vi "PPMS Monitor and Control.vi"() -> ()   [LabVIEW 2016, in "instrument.PPMS2.lvclass"]
doc: "This VI will launch the PPMS 2 Instrument backend that will contunously monitor the state of the instrument and log to the DSC. The user has the option of launching a user interface (default) or allowing the backend to run headless. Run \"Launch PPMS2 UI.vi\" here or on a different computer to have a remote user interface. You can also use the APIs like \"Get Temperturature\" interact programmatically with the PPMS 2 Instrument backend."
uses:
  instrument.PPMS2.lvclass
  <vilib>/JKI/JKI SMO/SMO/Typedefs/SMOState --Enum.ctl
  C:/Program Files (x86)/National Instruments/LabVIEW 2016/vi.lib/JKI/JKI SMO/SMO/SMO.lvclass
  instrument.PPMS2 UI/Instrument.PPMS2 UI.lvclass
  C:/Program Files (x86)/National Instruments/LabVIEW 2016/vi.lib/JKI/JKI SMO/SMO.UI/SMO.UI.lvclass
  <vilib>/JKI/JKI SMO/SMO/SMO.lvclass
  <vilib>/JKI/JKI SMO/SMO.UI/SMO.UI.lvclass
panel:
  in  "Start UI?":bool=TRUE
  in  "Stop":bool=TRUE
  in  "Start":bool=TRUE
  in  "Splash Status":string="Push Start to Start..." caption="String"
  out "UI SMO State":T1=enum."Stopped"
  out "SMO State":T1
  out "error out":errorcluster
  # "PPMS Monitor and Control.vi"
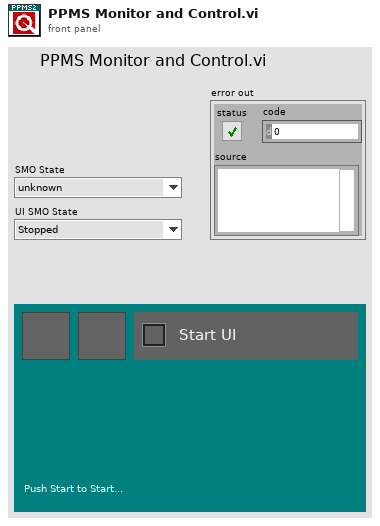
[diagram p1: front panel]
types:
  T1 = typedef "SMO.lvclass/SMOState --Enum.ctl" = enum16{"unknown", "Created", "Started", "Stopped"}
  T2 = enum32{"Invalid", "Standard", "Closed", "Hidden", "Minimized", "Maximized"}
  T3 = typedef "SMO.lvclass/Public Events.ctl" = cluster{"Error":refnum<user-event>, "State":refnum<user-event>, "Reserve State":refnum<user-event>}
  T4 = cluster{"Event Registration Refnum":refnum<event-registration>, "Event Registration Refnum":refnum<event-registration>}
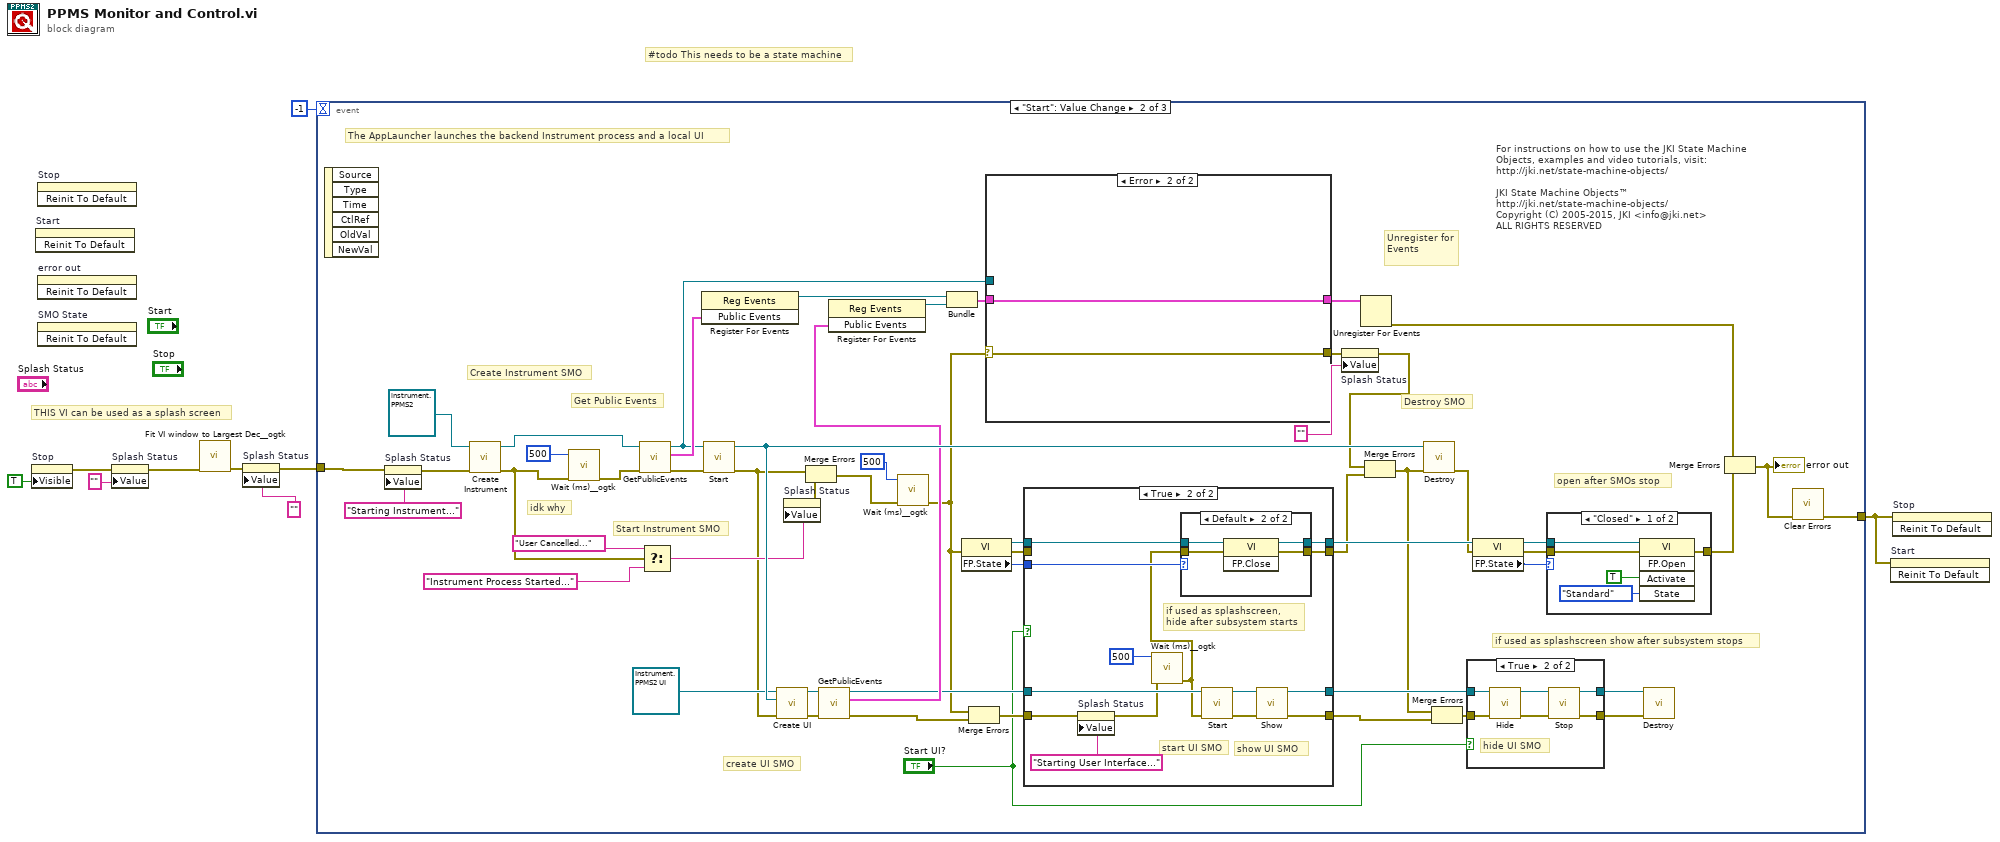
[diagram p0: block diagram]
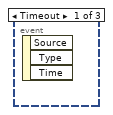
[diagram p2: hidden frame]
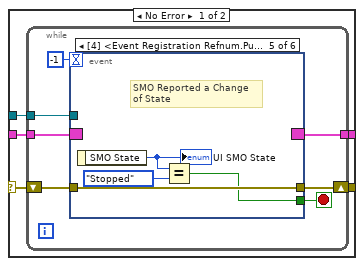
[diagram p3: hidden frame]
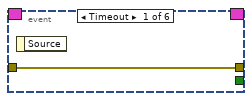
[diagram p4: hidden frame]
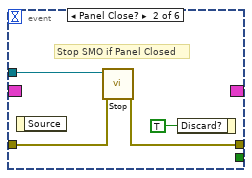
[diagram p5: hidden frame]
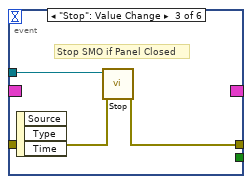
[diagram p6: hidden frame]
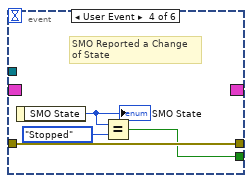
[diagram p7: hidden frame]
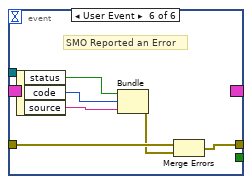
[diagram p8: hidden frame]
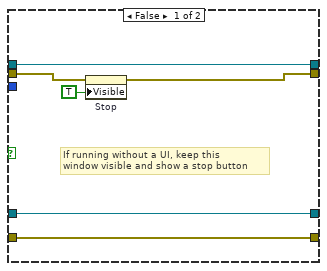
[diagram p10: hidden frame]
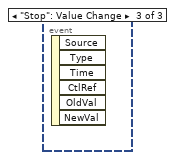
[diagram p13: hidden frame]
diagram:
  # "#todo This needs to be a state machine"
  # "THIS VI can be used as a splash screen"
  n1 = property on="Stop" class="Bool (strict)"("Visible"=TRUE) -> (error out=w7:errorcluster)  [unwired: 2 in, 1 out]
  n2 = invoke on="Start" class="Bool (strict)" method="Reinit To Default"() -> ()  [unwired: 3 in, 3 out]
  n3 = invoke on="Stop" class="Bool (strict)" method="Reinit To Default"() -> ()  [unwired: 3 in, 3 out]
  n4 = invoke on="error out" class="Clust (strict)" method="Reinit To Default"() -> ()  [unwired: 3 in, 3 out]
  n5 = invoke on="SMO State" class="Enum (strict)" method="Reinit To Default"() -> ()  [unwired: 3 in, 3 out]
  n6 = property on="Splash Status" class="Str"(error in=w7, "Value"="" ("Splash Status")) -> (error out=w9:errorcluster)  [unwired: 1 in, 1 out]
  n7 = call <userlib>:"Fit VI window to Largest Dec__ogtk.vi"("error in (no error)"=w9) -> ("error out"=w4:errorcluster)  [unwired: 5 in, 1 out]
  n8 = property on="Splash Status" class="Str"(error in=w4, "Value"="" ("Splash Status")) -> (error out=w3:errorcluster)  [unwired: 1 in, 1 out]
  n9 = event shown="[1] \"Start\": Value Change" {
    selector: _ -> [_ _ _]
    dyn-events: _ -> [_ _ _]
    timeout: -1 -> [_ _ _]
    tunnel: w3 -> [_ w21 _]
    tunnel: [_ w17 _] -> w1
    event Timeout {
      n10 = event-data() -> ()  [unwired: 1 in, 3 out]
    }
    event "Start": Value Change {
      # "idk why"
      # "open after SMOs stop"
      # "create UI SMO"
      # "if used as splashscreen show after subsystem stops"
      # "The AppLauncher launches the backend Instrument process and a local UI"
      # "Get Public Events"
      # "Start Instrument SMO"
      # "Destroy SMO"
      # "Create Instrument SMO"
      # "Unregister for Events"
      # "For instructions on how to use the JKI State Machine Objects, examples and video tutorials, visit:\nhttp://jki.net/state-machine-objects/\n\nJKI State Machine Objects™\nhttp://jki.net/state-machine-objects/\nCopyright (C) 2005-2015, JKI <info@jki.net>\nALL RIGHTS RESERVED"
      n11 = event-data() -> ()  [unwired: 1 in, 6 out]
      n12 = property on="Splash Status" class="Str"(error in=w21, "Value"="Starting Instrument..." ("Splash Status")) -> (error out=w30:errorcluster)  [unwired: 1 in, 1 out]
      n13 = call-dynamic "Create Instrument.vi"("error in (no error)"=w30, "Instrument in"=refnum<class "instrument.PPMS2.lvclass"> refnum ("SMO.Template.lvclass")) -> ("error out"=w16:errorcluster, "Instrument out"=w31:refnum<class "instrument.PPMS2.lvclass">)  [unwired: 8 in]
      n14 = call <userlib>:"Wait (ms)__ogtk.vi"("error in (no error)"=w16, "milliseconds to wait"=u32 500) -> ("error out"=w33:errorcluster)  [unwired: 8 in, 1 out]
      n15 = call <vilib>:"GetPublicEvents.vi"("error in (no error)"=w33, "SMO"=w31) -> ("error out"=w59:errorcluster, "Public Events"=w61:T3, "SMO out"=w60:refnum<class "instrument.PPMS2.lvclass">)  [unwired: 7 in]
      n16 = Select(t="User Cancelled...", s=w16, f="Instrument Process Started..." ("Splash Status")) -> (s? t:f=w15:string)
      n17 = register-events(w61) -> (reference out=w19:refnum<event-registration>)  [unwired: 2 in, 1 out]
      n18 = call <vilib>:"Start.vi"("error in (no error)"=w59, "SMO"=w60) -> ("error out"=w14:errorcluster, "SMO out"=w53:refnum<class "instrument.PPMS2.lvclass">)  [unwired: 8 in]
      n19 = call "Create UI.vi"("error in (no error)"=w14, "instrument.PPMS2"=w53, "Instrument.PPMS2 UI"=refnum<class "Instrument.PPMS2 UI.lvclass"> refnum ("SR7220 UI.lvclass")) -> ("error out"=w51:errorcluster, "Instrument.PPMS2 UI out"=w50:refnum<class "Instrument.PPMS2 UI.lvclass">)  [unwired: 7 in]
      n20 = property on="Splash Status" class="Str"("Value"=w15) -> (error out=w13:errorcluster)  [unwired: 2 in, 1 out]
      n21 = Merge Errors(w14, w13) -> (w12:errorcluster)
      n22 = call <vilib>:"GetPublicEvents.vi"("error in (no error)"=w51, "SMO"=w50) -> ("error out"=w44:errorcluster, "Public Events"=w49:T3, "SMO out"=w45:refnum<class "Instrument.PPMS2 UI.lvclass">)  [unwired: 7 in]
      n23 = register-events(w49) -> (reference out=w52:refnum<event-registration>)  [unwired: 2 in, 1 out]
      n24 = call <userlib>:"Wait (ms)__ogtk.vi"("error in (no error)"=w12, "milliseconds to wait"=u32 500) -> ("error out"=w18:errorcluster)  [unwired: 8 in, 1 out]
      n25 = Bundle("Event Registration Refnum"=w19, "Event Registration Refnum"=w52) -> (w54:T4)  [unwired: 1 in]
      n26 = property class="VI"(error in=w18) -> (reference out=w39:refnum<vi>, error out=w40:errorcluster, "FP.State"=w38:T2)  [unwired: 1 in]
      n27 = Merge Errors(w18, w44) -> (w48:errorcluster)
      n28 = case shown="Error" w18 {
        selector: w18 -> [w64 w99]
        tunnel: [w68 w98] -> w63
        tunnel: w60 -> [w67 _]
        tunnel: w54 -> [w66 w98]
        tunnel: [w65 w99] -> w27
        frame No Error {
          n29 = while {
            shift-right: [w74] -> w65
            shift-left: w64 -> [w73]
            tunnel: w66 -> [w72]
            tunnel: [w71] -> w68
            tunnel: w67 -> [w70]
            stop <- w75 stop-if-true
            n30 = event shown="[4] <Event Registration Refnum.Public Events.State>: User Event" {
              selector: w72 -> [_ _ _ _ _ _]
              dyn-events: [_ _ _ _ _ _] -> w71
              timeout: -1 -> [_ _ _ _ _ _]
              tunnel: [_ _ _ w84 w88 _] -> w75
              tunnel: w70 -> [_ w80 w83 _ _ _]
              tunnel: [w76 w79 w82 w87 w91 w92] -> w74
              tunnel: w73 -> [w76 w78 w81 w87 w91 w94]
              event Timeout {
                n31 = event-data() -> ()  [unwired: 1 in, 1 out]
              }
              event Panel Close? {
                # "Stop SMO if Panel Closed"
                n32 = event-data() -> ()  [unwired: 1 in, 1 out]
                n33 = call <vilib>:"Stop.vi"("error in (no error)"=w78, "SMO"=w80) -> ("error out"=w79:errorcluster)  [unwired: 8 in, 1 out]
                n34 = event-data("Discard?"=TRUE ("OK")) -> ()  [unwired: 1 in, 1 out]
              }
              event "Stop": Value Change {
                # "Stop SMO if Panel Closed"
                n35 = event-data() -> ()  [unwired: 1 in, 3 out]
                n36 = call <vilib>:"Stop.vi"("error in (no error)"=w81, "SMO"=w83) -> ("error out"=w82:errorcluster)  [unwired: 8 in, 1 out]
              }
              event User Event {
                # "SMO Reported a Change\nof State"
                n37 = event-data() -> ("SMO State"=w86:T1)  [unwired: 1 in]
                "SMO State" <- w86
                n38 = Equal?(x=w86, y=SMOState_--Enum."Stopped") -> (x = y?=w84:bool)
              }
              event User Event {
                # "SMO Reported a Change\nof State"
                n39 = event-data() -> ("SMO State"=w90:T1)  [unwired: 1 in]
                "UI SMO State" <- w90
                n40 = Equal?(x=w90, y=SMOState_--Enum."Stopped") -> (x = y?=w88:bool)
              }
              event User Event {
                # "SMO Reported an Error"
                n41 = event-data() -> ("status"=w95:bool, "code"=w97:i32, "source"=w96:string)  [unwired: 1 in]
                n42 = Bundle("status"=w95, "code"=w97, "source"=w96) -> (w93:errorcluster)  [unwired: 1 in]
                n43 = Merge Errors(w94, w93) -> (w92:errorcluster)
              }
            }
          }
        }
        frame Error {
        }
      }
      n44 = case shown="True" "Start UI?" {
        tunnel: [w111 w127] -> w58
        tunnel: [w112 w126] -> w55
        tunnel: w48 -> [w108 w118]
        tunnel: w45 -> [w109 w125]
        tunnel: [w109 w122] -> w42
        tunnel: w40 -> [w110 _]
        tunnel: w39 -> [w111 w121]
        tunnel: w38 -> [_ w120]
        tunnel: [w108 w119] -> w28
        frame False {
          # "If running without a UI, keep this\nwindow visible and show a stop button"
          n45 = property on="Stop" class="Bool (strict)"(error in=w110, "Visible"=TRUE) -> (error out=w112:errorcluster)  [unwired: 1 in, 1 out]
        }
        frame True {
          # "show UI SMO"
          # "start UI SMO"
          # "if used as splashscreen,\nhide after subsystem starts"
          n46 = property on="Splash Status" class="Str"(error in=w118, "Value"="Starting User Interface..." ("Splash Status")) -> (error out=w116:errorcluster)  [unwired: 1 in, 1 out]
          n47 = call <userlib>:"Wait (ms)__ogtk.vi"("error in (no error)"=w116, "milliseconds to wait"=u32 500) -> ("error out"=w114:errorcluster)  [unwired: 8 in, 1 out]
          n48 = case shown="Default" w120 {
            tunnel: [w129 w133] -> w126
            tunnel: w114 -> [w129 w132]
            tunnel: w121 -> [w128 w131]
            tunnel: [w128 w130] -> w127
            frame "Invalid", "Closed" {
            }
            frame Default {
              n49 = invoke class="VI" method="FP.Close"(reference=w131, error in=w132) -> (reference out=w130:refnum<vi>, error out=w133:errorcluster)  [unwired: 1 in, 1 out]
            }
          }
          n50 = call <vilib>:"Start.vi"("error in (no error)"=w114, "SMO"=w125) -> ("error out"=w124:errorcluster, "SMO out"=w123:refnum<class "Instrument.PPMS2 UI.lvclass">)  [unwired: 8 in]
          n51 = call <vilib>:"Show.vi"("error in (no error)"=w124, "SMO.UI"=w123) -> ("error out"=w119:errorcluster, "SMO.UI out"=w122:refnum<class "Instrument.PPMS2 UI.lvclass">)  [unwired: 8 in]
        }
      }
      n52 = property on="Splash Status" class="Str"(error in=w27, "Value"="" ("Splash Status")) -> (error out=w26:errorcluster)  [unwired: 1 in, 1 out]
      n53 = Unregister For Events(event registration refnum=w63) -> (error out=w62:errorcluster)  [unwired: 1 in]
      n54 = Merge Errors(w26, w55) -> (w29:errorcluster)
      n55 = call <vilib>:"Destroy.vi"("error in (no error)"=w29, "SMO"=w53) -> ("error out"=w57:errorcluster)  [unwired: 9 in]
      n56 = Merge Errors(w29, w28) -> (w43:errorcluster)
      n57 = case shown="True" "Start UI?" {
        tunnel: [w101 w107] -> w47
        tunnel: [w100 w106] -> w46
        tunnel: w43 -> [w101 w103]
        tunnel: w42 -> [w100 w102]
        frame False {
        }
        frame True {
          # "hide UI SMO"
          n58 = call <vilib>:"Hide.vi"("error in (no error)"=w103, "SMO.UI"=w102) -> ("error out"=w105:errorcluster, "SMO.UI out"=w104:refnum<class "Instrument.PPMS2 UI.lvclass">)  [unwired: 8 in]
          n59 = call <vilib>:"Stop.vi"("error in (no error)"=w105, "SMO"=w104) -> ("error out"=w107:errorcluster, "SMO out"=w106:refnum<class "Instrument.PPMS2 UI.lvclass">)  [unwired: 8 in]
        }
      }
      n60 = property class="VI"(reference=w58, error in=w57) -> (reference out=w36:refnum<vi>, error out=w37:errorcluster, "FP.State"=w35:T2)
      n61 = case shown="\"Closed\"" w35 {
        tunnel: [w136 w139] -> w56
        tunnel: w37 -> [w135 w139]
        tunnel: w36 -> [w134 _]
        frame "Closed" {
          n62 = invoke class="VI" method="FP.Open"(reference=w134, error in=w135, "Activate"=TRUE, "State"=T2."Standard") -> (error out=w136:errorcluster)  [unwired: 1 in, 4 out]
        }
        frame Default {
        }
      }
      n63 = call <vilib>:"Destroy.vi"("error in (no error)"=w47, "SMO"=w46) -> ()  [unwired: 9 in, 1 out]
      n64 = Merge Errors(w62, w56) -> (w20:errorcluster)
      "error out" <- w20
      n65 = call <vilib>:"Clear Errors.vi"("error in (no error)"=w20) -> ("error out"=w17:errorcluster)  [unwired: 5 in, 1 out]
    }
    event "Stop": Value Change {
      n66 = event-data() -> ()  [unwired: 1 in, 6 out]
    }
  }
  n67 = invoke on="Start" class="Bool (strict)" method="Reinit To Default"(error in=w1) -> ()  [unwired: 2 in, 3 out]
  n68 = invoke on="Stop" class="Bool (strict)" method="Reinit To Default"(error in=w1) -> ()  [unwired: 2 in, 3 out]
